vi "Main_Module.vi"(11 "Error_In":errorcluster) -> (15 "Error_Out":errorcluster)   [LabVIEW 2023]
doc: "This is the Main VI that simulates the ADQ system. Captures the data generated in Data acquisition VI and send it to Logger VI to log the Errors."
uses:
  Controls/Current_Limit.ctl
  Controls/Temperature_Limit.ctl
  Controls/DAQ_Data.ctl
  Controls/State_and_Data.ctl
  Controls/Queue_Operation_Select.ctl
  Controls/Notifier_Operation_Select.ctl
panel:
  in  "Logging_Rate":u32=1 caption="Logging Rate"
  in  "Exit":bool
  in  "Acquisition":bool
  in  "Temperature_Limit":T1={"Temperature_High_Limit"=50.0, "Temperature_Low_Limit"=30.0} caption="Temperature Limit" {"Temperature_Low_Limit" min=30.0 max=49.0; "Temperature_High_Limit" min=31.0 max=50.0}
  in  "Current_Limit":T2={"Current_High_Limit"=120.0, "Current_Low_Limit"=100.0} caption="Current Limit" {"Current_High_Limit" min=101.0 max=120.0; "Current_Low_Limit" min=100.0 max=119.0}
  out "Temperature":dbl
  out "Current":dbl
  out "Generated_Data":dbl[][](graph)
  # "DAQ System"
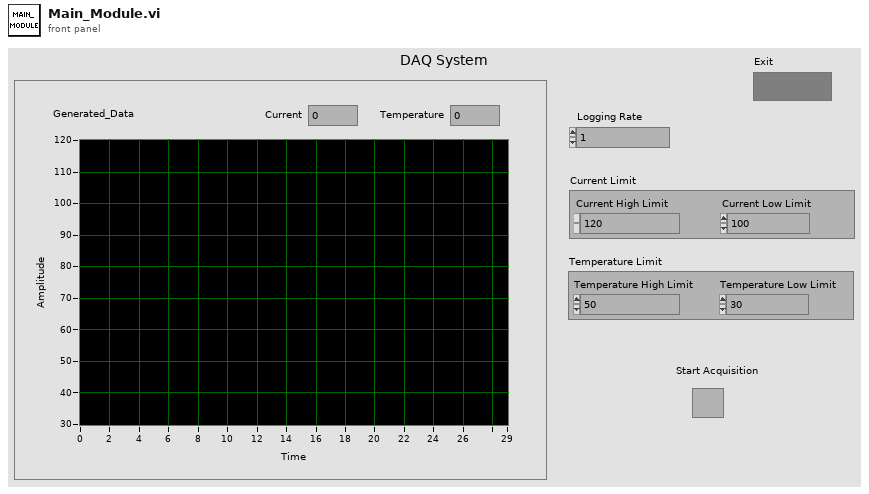
[diagram p1: front panel]
types:
  T1 = typedef "Temperature_Limit.ctl" = cluster{"Temperature_High_Limit":dbl, "Temperature_Low_Limit":dbl}
  T2 = typedef "Current_Limit.ctl" = cluster{"Current_High_Limit":dbl, "Current_Low_Limit":dbl}
  T3 = typedef "Queue_Operation_Select.ctl" = enum16{"Obtain_Queue", "Enqueue", "Enqueue_First", "Enqueue_N", "Lossy_Enqueue", "Preview", "Queue_Status", "Dequeue", "Flush", "Release_Queue"}
  T4 = typedef "Notifier_Operation_Select.ctl" = enum16{"Obtain_Notifier", "Send_Notification", "Get_Notifier_Status", "Release_Notifier"}
  T5 = typedef "State_and_Data.ctl" = cluster{"State":string, "Data":variant}
  T6 = typedef "DAQ_Data.ctl" = cluster{"Wait_Time":dbl, "Start/Stop_Acquisition ":bool, "Generated_Data ":dbl[][], "Current":dbl, "Temperature":dbl, "Disabled":enum8{"Enabled", "Disabled", "Disabled and Grayed Out"}, "Temperature_Limit":T1, "Current_Limit":T2, "State_and_Data_In":T5}
  T7 = enum8{"Enabled", "Disabled", "Disabled and Grayed Out"}
  T8 = typedef "Generated_data.ctl" = cluster{"Current_Data":dbl, "Temp_Data":dbl}
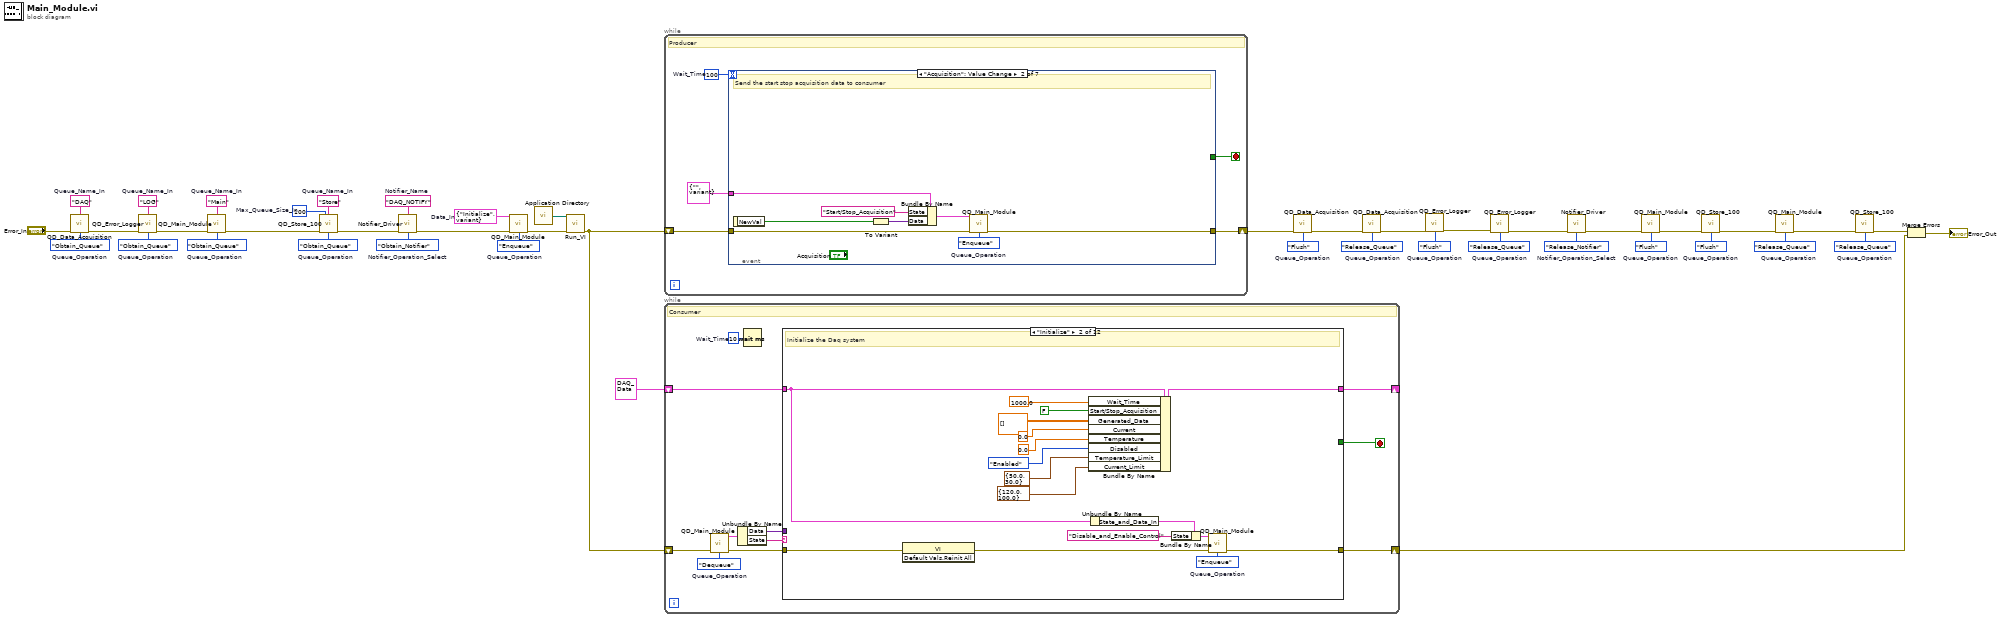
[diagram p0: block diagram]
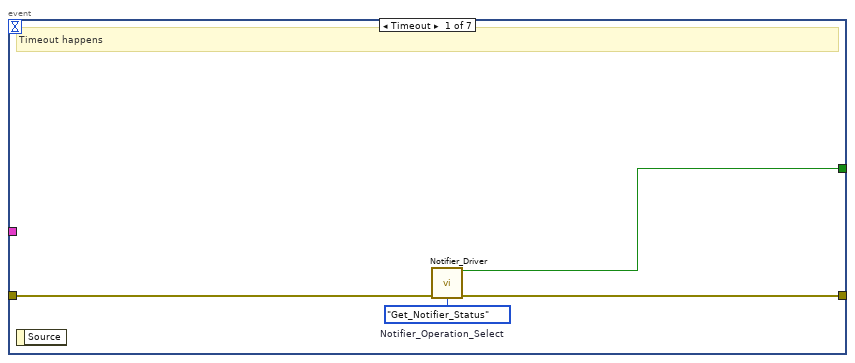
[diagram p2: hidden frame]
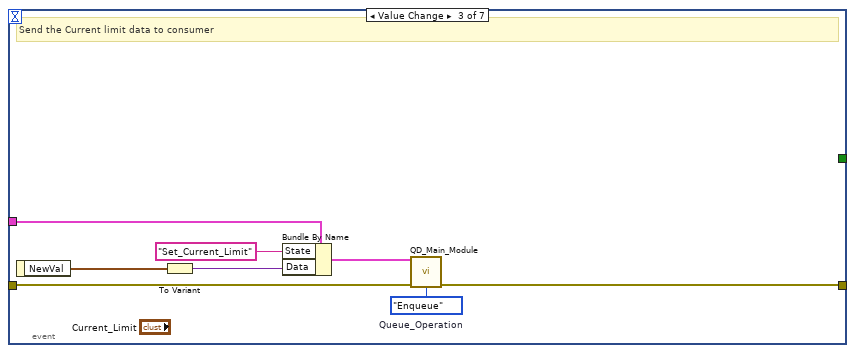
[diagram p3: hidden frame]
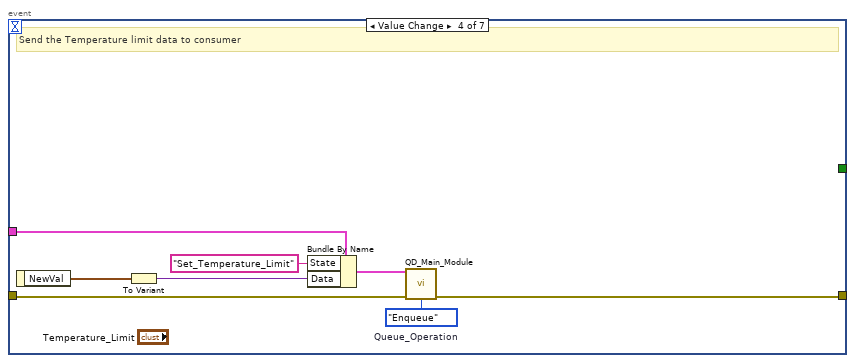
[diagram p4: hidden frame]
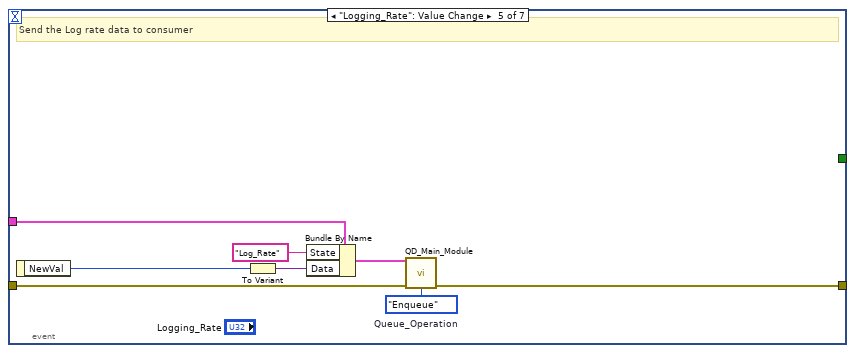
[diagram p5: hidden frame]
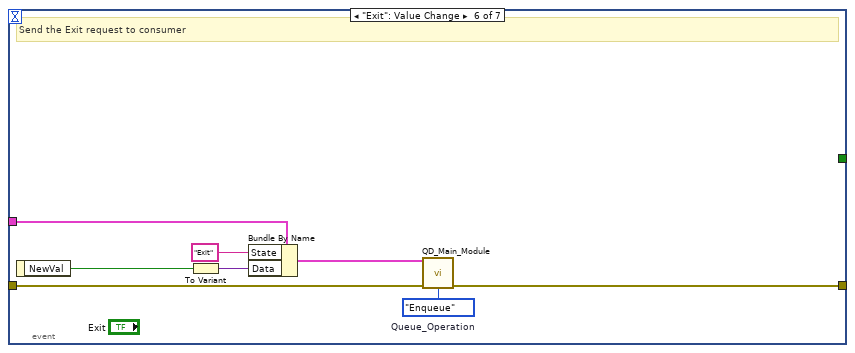
[diagram p6: hidden frame]
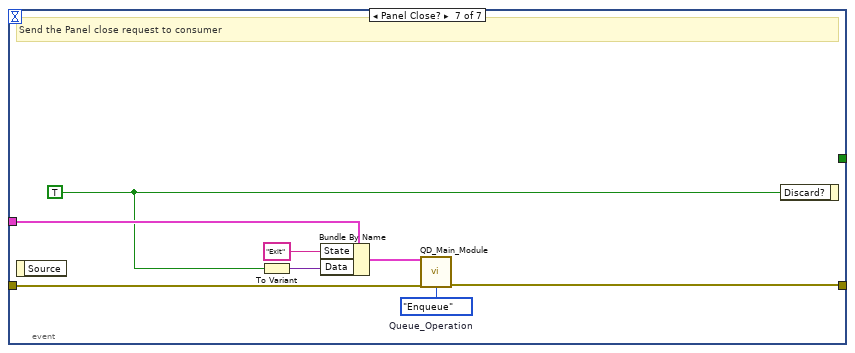
[diagram p7: hidden frame]
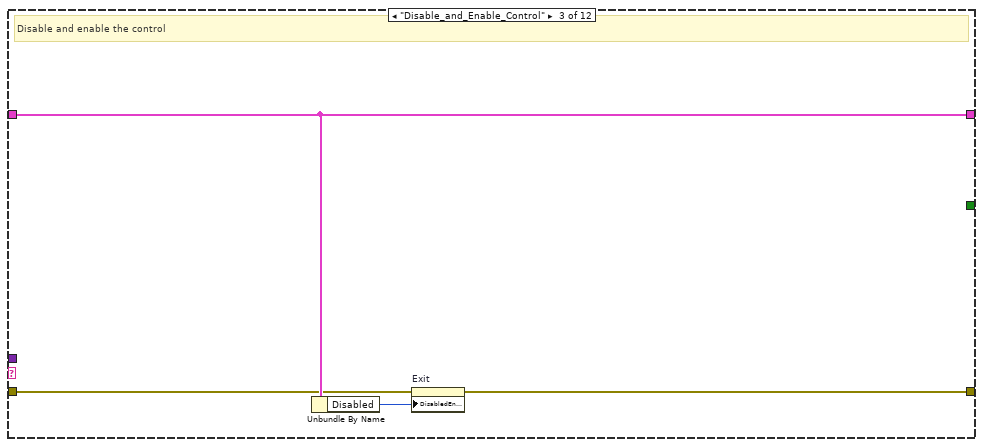
[diagram p9: hidden frame]
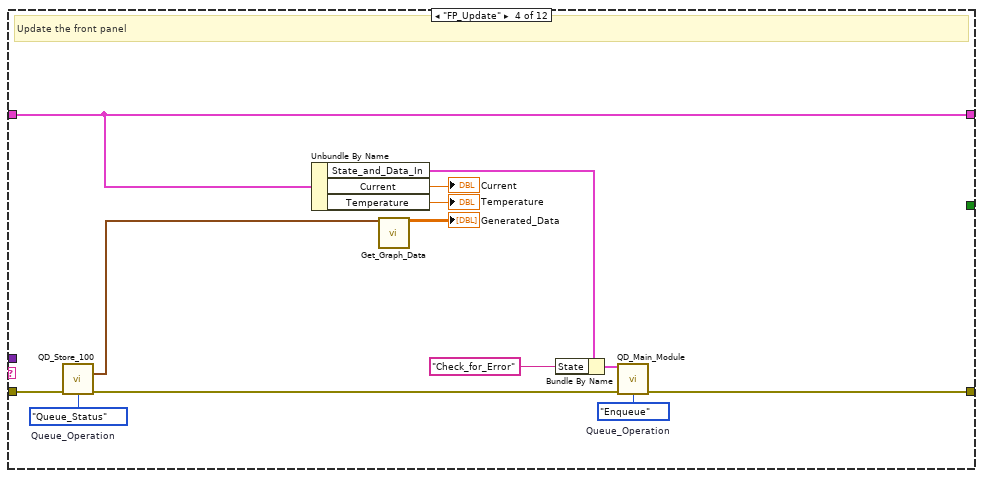
[diagram p10: hidden frame]
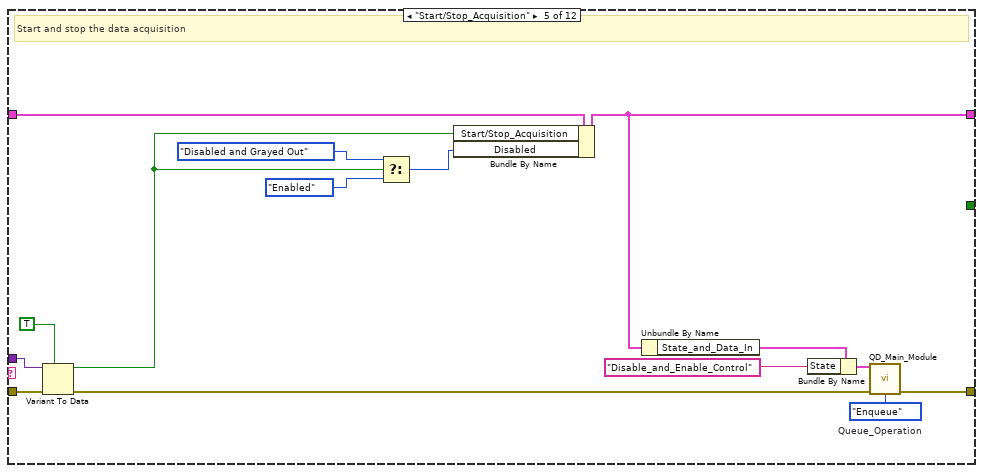
[diagram p11: hidden frame]
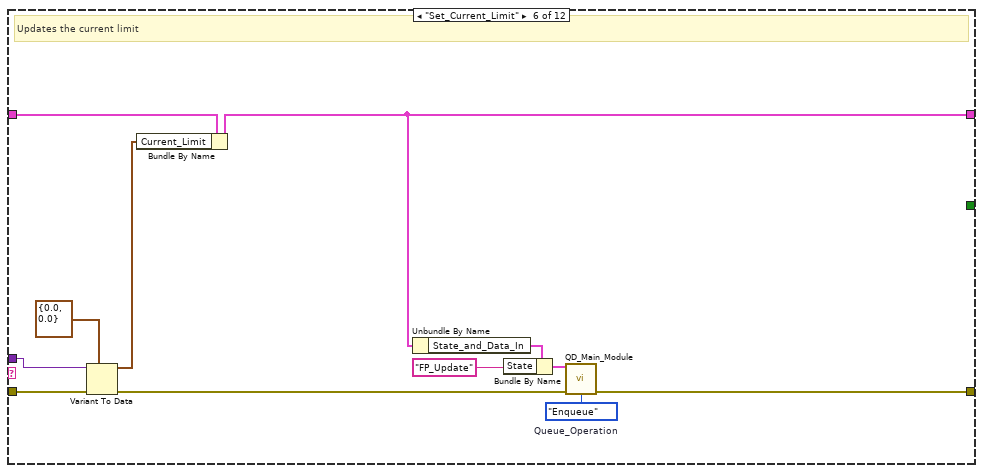
[diagram p12: hidden frame]
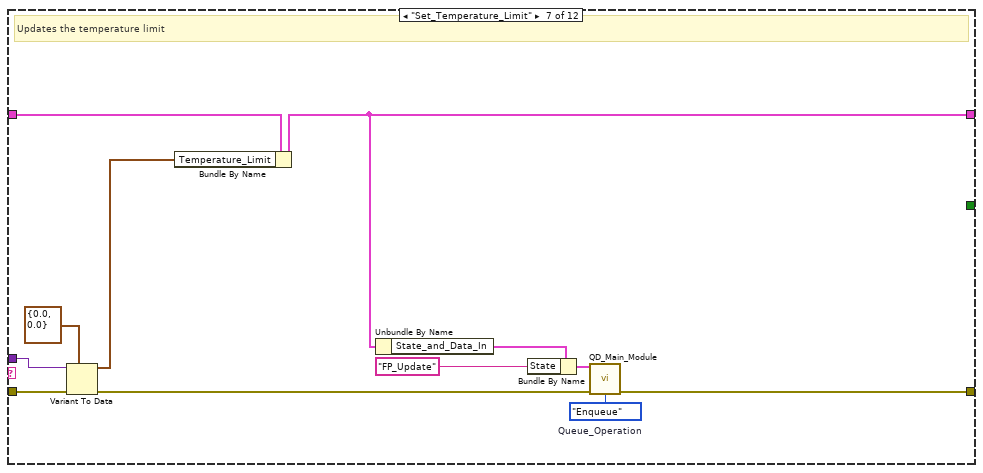
[diagram p13: hidden frame]
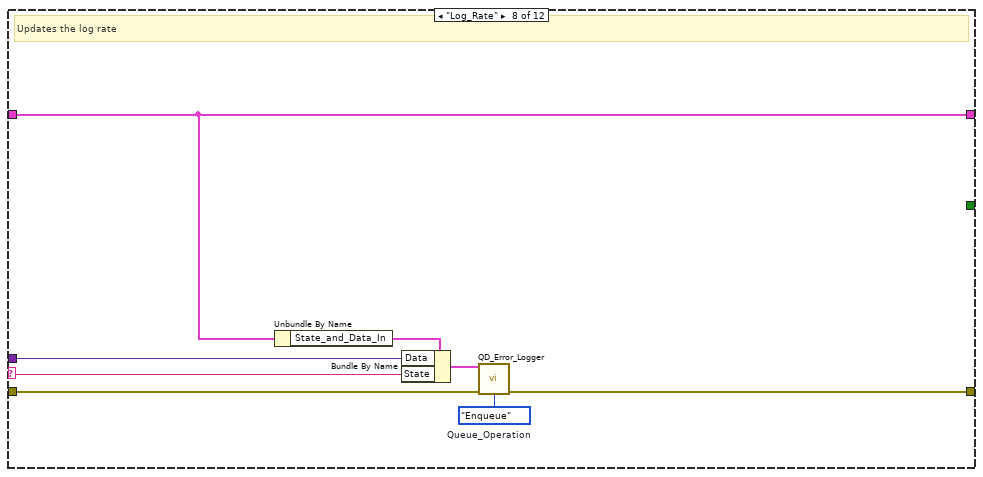
[diagram p14: hidden frame]
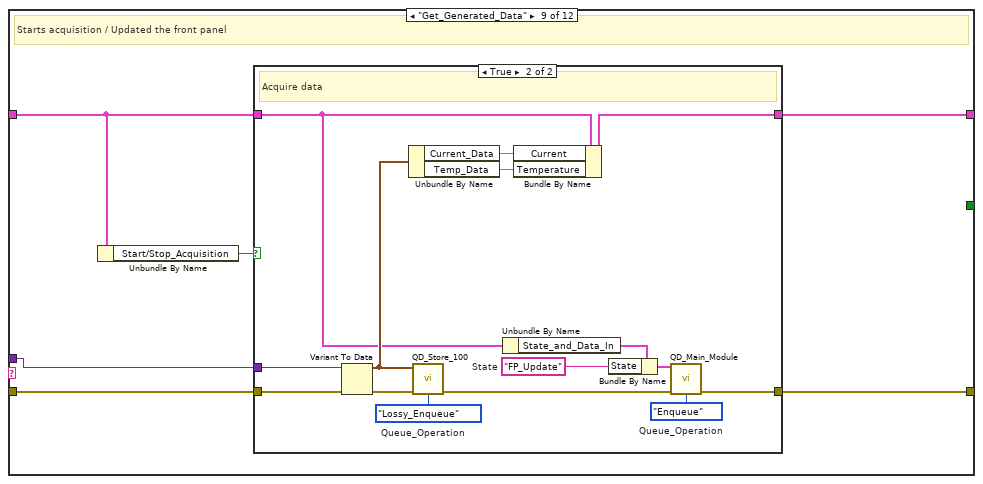
[diagram p15: hidden frame]
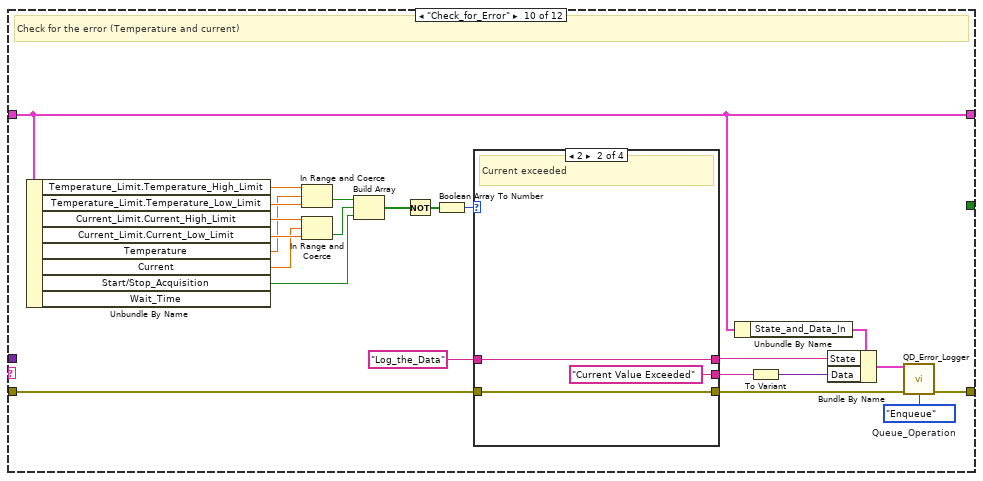
[diagram p17: hidden frame]
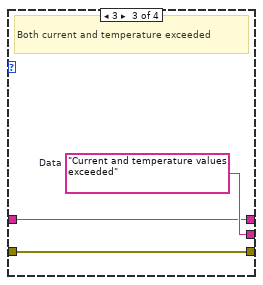
[diagram p19: hidden frame]
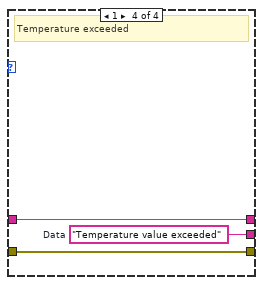
[diagram p20: hidden frame]
diagram:
  w3 = Queue_Operation_Select."Release_Queue"  # Queue_Operation
  w4 = Queue_Operation_Select."Flush"  # Queue_Operation
  w5 = "DAQ_NOTIFY"  # Notifier_Name
  w14 = Notifier_Operation_Select."Release_Notifier"  # Notifier_Operation_Select
  w15 = Queue_Operation_Select."Flush"  # Queue_Operation
  w16 = Queue_Operation_Select."Flush"  # Queue_Operation
  w17 = Queue_Operation_Select."Release_Queue"  # Queue_Operation
  w18 = Queue_Operation_Select."Release_Queue"  # Queue_Operation
  w20 = Queue_Operation_Select."Release_Queue"  # Queue_Operation
  w21 = Queue_Operation_Select."Flush"  # Queue_Operation
  w22 = Notifier_Operation_Select."Obtain_Notifier"  # Notifier_Operation_Select
  w24 = T5 {"State"="Initialize", "Data"=variant}  # Data_In
  w27 = Queue_Operation_Select."Enqueue"  # Queue_Operation
  w29 = "Store"  # Queue_Name_In
  w30 = "Main"  # Queue_Name_In
  w31 = Queue_Operation_Select."Obtain_Queue"  # Queue_Operation
  w33 = "LOG"  # Queue_Name_In
  w34 = "DAQ"  # Queue_Name_In
  w40 = Queue_Operation_Select."Obtain_Queue"  # Queue_Operation
  w41 = Queue_Operation_Select."Obtain_Queue"  # Queue_Operation
  w38 = 100  # Max_Queue_Size_In
  w43 = Queue_Operation_Select."Obtain_Queue"  # Queue_Operation
  n1 = call "QD_Data_Acquisition.vi"("Queue_Name_In"=w34, "Error_In"="Error_In", "Queue_Operation"=w43) -> ("Error_Out"=w44:errorcluster)  [unwired: 10 in, 2 out]
  n2 = call "QD_Error_Logger.vi"("Queue_Name_In"=w33, "Error_In"=w44, "Queue_Operation"=w41) -> ("Error_Out"=w42:errorcluster)  [unwired: 11 in, 1 out]
  n3 = call "QD_Main_Module.vi"("Queue_Name_In"=w30, "Error_In"=w42, "Queue_Operation"=w31) -> ("Error_Out"=w32:errorcluster)  [unwired: 10 in, 2 out]
  n4 = call "QD_Store_100.vi"("Max_Queue_Size_In"=w38, "Queue_Name_In"=w29, "Error_In"=w32, "Queue_Operation"=w40) -> ("Error_Out"=w37:errorcluster)  [unwired: 9 in, 2 out]
  n5 = call "Notifier_Driver.vi"("Notifier_Name"=w5, "Error_In"=w37, "Notifier_Operation_Select"=w22) -> ("Error_Out"=w23:errorcluster)  [unwired: 11 in, 1 out]
  n6 = call "QD_Main_Module.vi"("Data_In"=w24, "Error_In"=w23, "Queue_Operation"=w27) -> ("Error_Out"=w28:errorcluster)  [unwired: 10 in, 2 out]
  n7 = call <vilib>:"Application Directory.vi"() -> ("Application Directory"=w39:path)
  n8 = call "Run_VI.vi"("Application_Directory"=w39, "Error_In"=w28) -> ("Error_Out"=w26:errorcluster)  [unwired: 13 in]
  n9 = while {
    shift-right: [w55] -> _
    shift-left: T6 {"Wait_Time"=1000.0, "Start/Stop_Acquisition "=FALSE, "Generated_Data "=[], "Current"=0.0, "Temperature"=0.0, "Disabled"=enum."Enabled", "Temperature_Limit"={"Temperature_High_Limit"=0.0, "Temperature_Low_Limit"=0.0}, "Current_Limit"={"Current_High_Limit"=101.0, "Current_Low_Limit"=100.0}, "State_and_Data_In"={"State"="", "Data"=variant}} -> [w47]
    shift-right: [w45] -> w25
    shift-left: w26 -> [w54]
    stop <- w48 stop-if-true
    w46 = u32 10  # Wait_Time
    w52 = Queue_Operation_Select."Dequeue"  # Queue_Operation
    # "Consumer"
    n10 = call "QD_Main_Module.vi"("Error_In"=w54, "Queue_Operation"=w52) -> ("Data_Out"=w51:T5, "Error_Out"=w53:errorcluster)  [unwired: 11 in, 1 out]
    n11 = Unbundle By Name(w51) -> ("Data"=w49:variant, "State"=w50:string)
    n12 = Wait (ms)(milliseconds to wait=w46) -> ()  [unwired: 1 out]
    n13 = case shown="\"Initialize\"" w50 {
      selector: w50 -> [_ _ _ _ _ _ _ w135 _ _ _ _]
      tunnel: w53 -> [w56 w74 w77 w85 w106 w118 w130 w138 w144 w171 w204 w224]
      tunnel: w47 -> [w57 w61 w78 w91 w96 w111 w123 w133 w142 w164 w197 w225]
      tunnel: [w57 w73 w78 w91 w92 w110 w121 w133 w140 w164 w197 w225] -> w55
      tunnel: w49 -> [_ _ _ _ w105 w117 w129 w137 w143 _ _ _]
      tunnel: [_ _ _ _ _ _ _ _ _ _ _ w215] -> w48
      tunnel: [w56 w58 w75 w79 w93 w107 w119 w131 w139 w162 w195 w214] -> w45
      frame Default {
        # "Nothing will be done here"
      }
      frame "Initialize" {
        w64 = Queue_Operation_Select."Enqueue"  # Queue_Operation
        # "Initialize the Daq system"
        n14 = invoke class="VI" method="Default Vals.Reinit All"(error in=w74) -> (error out=w62:errorcluster)  [unwired: 2 in, 2 out]
        n15 = Bundle By Name(cluster=w61, "Wait_Time"=1000.0, "Start/Stop_Acquisition"=FALSE, "Generated_Data"=dbl[][] [], "Current"=0.0, "Temperature"=0.0, "Disabled"=T7."Enabled", "Temperature_Limit"=T1 {"Temperature_High_Limit"=50.0, "Temperature_Low_Limit"=30.0}, "Current_Limit"=T2 {"Current_High_Limit"=120.0, "Current_Low_Limit"=100.0}) -> (w73:T6)
        n16 = Unbundle By Name(w61) -> ("State_and_Data_In"=w60:T5)
        n17 = Bundle By Name(cluster=w60, "State"="Disable_and_Enable_Control") -> (w63:T5)
        n18 = call "QD_Main_Module.vi"("Data_In"=w63, "Error_In"=w62, "Queue_Operation"=w64) -> ("Error_Out"=w58:errorcluster)  [unwired: 10 in, 2 out]
      }
      frame "Disable_and_Enable_Control" {
        # "Disable and enable the control"
        n19 = Unbundle By Name(w78) -> ("Disabled"=w76:T7)
        n20 = property on="Exit" class="Bool (strict)"(error in=w77, "DisabledEnum"=w76) -> (error out=w75:errorcluster)  [unwired: 1 in, 1 out]
      }
      frame "FP_Update" {
        w84 = Queue_Operation_Select."Enqueue"  # Queue_Operation
        w88 = Queue_Operation_Select."Queue_Status"  # Queue_Operation
        # "Update the front panel"
        n21 = call "QD_Store_100.vi"("Error_In"=w85, "Queue_Operation"=w88) -> ("Total_Data"=w86:T8[], "Error_Out"=w82:errorcluster)  [unwired: 11 in, 1 out]
        n22 = Unbundle By Name(w91) -> ("State_and_Data_In"=w81:T5, "Current"=→"Current":dbl, "Temperature"=→"Temperature":dbl)
        n23 = call "Get_Graph_Data.vi"("Total_Data"=w86) -> ("Array"=→"Generated_Data":dbl[][])  [unwired: 14 in]
        n24 = Bundle By Name(cluster=w81, "State"="Check_for_Error") -> (w83:T5)
        n25 = call "QD_Main_Module.vi"("Data_In"=w83, "Error_In"=w82, "Queue_Operation"=w84) -> ("Error_Out"=w79:errorcluster)  [unwired: 10 in, 2 out]
      }
      frame "Start/Stop_Acquisition" {
        w99 = Queue_Operation_Select."Enqueue"  # Queue_Operation
        # "Start and stop the data acquisition"
        n26 = Variant To Data(error in=w106, type=TRUE, Variant=w105) -> (data=w101:bool, error out=w97:errorcluster)
        n27 = Select(t=T7."Disabled and Grayed Out", s=w101, f=T7."Enabled" ("Disabled")) -> (s? t:f=w103:T7)
        n28 = Bundle By Name(cluster=w96, "Start/Stop_Acquisition"=w101, "Disabled"=w103) -> (w92:T6)
        n29 = Unbundle By Name(w92) -> ("State_and_Data_In"=w95:T5)
        n30 = Bundle By Name(cluster=w95, "State"="Disable_and_Enable_Control") -> (w98:T5)
        n31 = call "QD_Main_Module.vi"("Data_In"=w98, "Error_In"=w97, "Queue_Operation"=w99) -> ("Error_Out"=w93:errorcluster)  [unwired: 10 in, 2 out]
      }
      frame "Set_Current_Limit" {
        w112 = Queue_Operation_Select."Enqueue"  # Queue_Operation
        # "Updates the current limit"
        n32 = Variant To Data(error in=w118, type=T2 {"Current_High_Limit"=0.0, "Current_Low_Limit"=0.0} ("Current_Limit"), Variant=w117) -> (data=w115:T2, error out=w113:errorcluster)
        n33 = Bundle By Name(cluster=w111, "Current_Limit"=w115) -> (w110:T6)
        n34 = Unbundle By Name(w110) -> ("State_and_Data_In"=w109:T5)
        n35 = Bundle By Name(cluster=w109, "State"="FP_Update") -> (w114:T5)
        n36 = call "QD_Main_Module.vi"("Data_In"=w114, "Error_In"=w113, "Queue_Operation"=w112) -> ("Error_Out"=w107:errorcluster)  [unwired: 10 in, 2 out]
      }
      frame "Set_Temperature_Limit" {
        w120 = Queue_Operation_Select."Enqueue"  # Queue_Operation
        # "Updates the temperature limit"
        n37 = Variant To Data(error in=w130, type=T1 {"Temperature_High_Limit"=0.0, "Temperature_Low_Limit"=0.0} ("Temperature_Limit"), Variant=w129) -> (data=w127:T1, error out=w125:errorcluster)
        n38 = Bundle By Name(cluster=w123, "Temperature_Limit"=w127) -> (w121:T6)
        n39 = Unbundle By Name(w121) -> ("State_and_Data_In"=w122:T5)
        n40 = Bundle By Name(cluster=w122, "State"="FP_Update") -> (w126:T5)
        n41 = call "QD_Main_Module.vi"("Data_In"=w126, "Error_In"=w125, "Queue_Operation"=w120) -> ("Error_Out"=w119:errorcluster)  [unwired: 10 in, 2 out]
      }
      frame "Log_Rate" {
        w134 = Queue_Operation_Select."Enqueue"  # Queue_Operation
        # "Updates the log rate"
        n42 = Unbundle By Name(w133) -> ("State_and_Data_In"=w132:T5)
        n43 = Bundle By Name(cluster=w132, "Data"=w137, "State"=w135) -> (w136:T5)
        n44 = call "QD_Error_Logger.vi"("State_and_Data_In"=w136, "Error_In"=w138, "Queue_Operation"=w134) -> ("Error_Out"=w131:errorcluster)  [unwired: 11 in, 1 out]
      }
      frame "Get_Generated_Data" {
        # "Starts acquisition / Updated the front panel"
        n45 = Unbundle By Name(w142) -> ("Start/Stop_Acquisition"=w141:bool)
        n46 = case shown="True" w141 {
          tunnel: w144 -> [w145 w160]
          tunnel: w142 -> [w146 w147]
          tunnel: w143 -> [_ w158]
          tunnel: [w146 w156] -> w140
          tunnel: [w145 w148] -> w139
          frame False {
          }
          frame True {
            w152 = Queue_Operation_Select."Enqueue"  # Queue_Operation
            w151 = "FP_Update"  # State
            w161 = Queue_Operation_Select."Lossy_Enqueue"  # Queue_Operation
            # "Acquire data"
            n47 = Variant To Data(error in=w160, Variant=w158) -> (data=w157:T8, error out=w159:errorcluster)  [unwired: 1 in]
            n48 = Unbundle By Name(w157) -> ("Current_Data"=w154:dbl, "Temp_Data"=w155:dbl)
            n49 = call "QD_Store_100.vi"("Generated_Data_In"=w157, "Error_In"=w159, "Queue_Operation"=w161) -> ("Error_Out"=w149:errorcluster)  [unwired: 10 in, 2 out]
            n50 = Unbundle By Name(w147) -> ("State_and_Data_In"=w150:T5)
            n51 = Bundle By Name(cluster=w147, "Current"=w154, "Temperature"=w155) -> (w156:T6)
            n52 = Bundle By Name(cluster=w150, "State"=w151) -> (w153:T5)
            n53 = call "QD_Main_Module.vi"("Data_In"=w153, "Error_In"=w149, "Queue_Operation"=w152) -> ("Error_Out"=w148:errorcluster)  [unwired: 10 in, 2 out]
          }
        }
      }
      frame "Check_for_Error" {
        w172 = Queue_Operation_Select."Enqueue"  # Queue_Operation
        # "Check for the error (Temperature and current)"
        n54 = Unbundle By Name(w164) -> ("Temperature_Limit.Temperature_High_Limit"=w184:dbl, "Temperature_Limit.Temperature_Low_Limit"=w183:dbl, "Current_Limit.Current_High_Limit"=w182:dbl, "Current_Limit.Current_Low_Limit"=w181:dbl, "Temperature"=w170:dbl, "Current"=w169:dbl, "Start/Stop_Acquisition"=w168:bool)  [unwired: 1 out]
        n55 = In Range and Coerce(upper limit=w184, x=w170, lower limit=w183) -> (In Range?=w166:bool)  [unwired: 1 out]
        n56 = In Range and Coerce(upper limit=w182, x=w169, lower limit=w181) -> (In Range?=w167:bool)  [unwired: 1 out]
        n57 = Build Array(w166, w167, w168) -> (w179:bool[])
        n58 = Not(x=w179) -> (.not. x?=w165:bool[])
        n59 = Boolean Array To Number(Boolean array=w165) -> (number=w178:u32)
        n60 = case shown="2" w178 {
          tunnel: [w185 w188 w191 w194] -> w180
          tunnel: w171 -> [w185 w188 w191 w194]
          tunnel: [_ "Current Value Exceeded" ("Data") w190 w193] -> w177
          tunnel: [_ w186 w189 w192] -> w174
          tunnel: "Log_the_Data" ("State") -> [_ w186 w189 w192]
          frame 0, Default {
          }
          frame 2 {
            # "Current exceeded"
          }
          frame 3 {
            w190 = "Current and temperature values exceeded"  # Data
            # "Both current and temperature exceeded"
          }
          frame 1 {
            w193 = "Temperature value exceeded"  # Data
            # "Temperature exceeded"
          }
        }
        n61 = Unbundle By Name(w164) -> ("State_and_Data_In"=w163:T5)
        n62 = To Variant(anything=w177) -> (Variant=w173:variant)
        n63 = Bundle By Name(cluster=w163, "State"=w174, "Data"=w173) -> (w175:T5)
        n64 = call "QD_Error_Logger.vi"("State_and_Data_In"=w175, "Error_In"=w180, "Queue_Operation"=w172) -> ("Error_Out"=w162:errorcluster)  [unwired: 11 in, 1 out]
      }
      frame "Error" {
        w209 = "%d%s%s"  # Format_String
        w210 = "Application Error"  # Initial_String
        w211 = "Stop"  # T_Button
        w212 = "Continue"  # F_Button
        # "Handles the appplication error"
        n65 = Unbundle By Name(w204) -> ("code"=w206:i32, "source"=w205:string)
        n66 = call <vilib>:"Clear Errors.vi"("error in (no error)"=w204) -> ("error out"=w207:errorcluster)  [unwired: 5 in, 1 out]
        n67 = Format Into String(format string=w209, initial string=w210, error in=w207, w206, "\n", w205) -> (resulting string=w213:string, error out=w199:errorcluster)
        n68 = Unbundle By Name(w197) -> ("State_and_Data_In"=w196:T5)
        n69 = Two Button Dialog(message=w213, 1:w212, 2:w211) -> (T button?=w202:bool)
        n70 = Select(t="Exit" ("State"), s=w202, f="") -> (s? t:f=w198:string)
        n71 = Bundle By Name(cluster=w196, "State"=w198) -> (w200:T5)
        n72 = call "QD_Main_Module.vi"("Data_In"=w200, "Error_In"=w199) -> ("Error_Out"=w195:errorcluster)  [unwired: 11 in, 2 out]
      }
      frame "Exit" {
        w218 = Notifier_Operation_Select."Send_Notification"  # Notifier_Operation_Select
        w219 = T5 {"State"="Exit", "Data"=variant}  # State_and_Data_In
        w220 = Queue_Operation_Select."Enqueue_First"  # Queue_Operation
        w221 = Queue_Operation_Select."Enqueue_First"  # Queue_Operation
        # "Exit the Application if the user wants to exit"
        n73 = disable-structure shown="Default" {
          disable-tunnel: [w226 w230] -> w215
          frame condition #0 (active) {
            w227 = "No"  # Back
            w228 = "Yes"  # Stop_Execution
            w229 = "Do you want to Stop the execution"  # Message
            # "Developer_Mode"
            n74 = Two Button Dialog(message=w229, 1:w227, 2:w228) -> (T button?=w226:bool)
          }
          frame condition #1 {
            w230 = TRUE  # Stop?
            # "Run_Time_Mode"
          }
        }
        n75 = Select(t=w219, s=w215, f=T5 {"State"="", "Data"=variant}) -> (s? t:f=w217:T5)
        n76 = call "QD_Error_Logger.vi"("State_and_Data_In"=w217, "Error_In"=w224, "Queue_Operation"=w221) -> ("Error_Out"=w223:errorcluster)  [unwired: 11 in, 1 out]
        n77 = call "QD_Data_Acquisition.vi"("State_and_Data_In"=w217, "Error_In"=w223, "Queue_Operation"=w220) -> ("Error_Out"=w222:errorcluster)  [unwired: 10 in, 2 out]
        n78 = call "Notifier_Driver.vi"("Notification"=w215, "Error_In"=w222, "Notifier_Operation_Select"=w218) -> ("Error_Out"=w214:errorcluster)  [unwired: 11 in, 1 out]
      }
    }
  }
  n79 = while {
    shift-right: [w231] -> w8
    shift-left: w26 -> [w235]
    stop <- w233 stop-if-true
    w234 = 100  # Wait_Time
    # "Producer"
    n80 = event shown="[1] \"Acquisition\": Value Change" {
      selector: _ -> [_ _ _ _ _ _ _]
      dyn-events: _ -> [_ _ _ _ _ _ _]
      timeout: w234 -> [_ _ _ _ _ _ _]
      tunnel: w235 -> [w236 w245 w253 w260 w271 w277 w283]
      tunnel: [w239 w244 w252 w259 w265 w276 w285] -> w231
      tunnel: [w237 _ _ _ _ _ _] -> w233
      tunnel: T5 {"State"="", "Data"=variant} ("Data_In") -> [_ w240 w249 w258 w266 w275 w284]
      event Timeout {
        w238 = Notifier_Operation_Select."Get_Notifier_Status"  # Notifier_Operation_Select
        # "Timeout happens"
        n81 = event-data() -> ()  [unwired: 1 in, 1 out]
        n82 = call "Notifier_Driver.vi"("Error_In"=w236, "Notifier_Operation_Select"=w238) -> ("Latest_Notification"=w237:bool, "Error_Out"=w239:errorcluster)  [unwired: 12 in]
      }
      event "Acquisition": Value Change {
        w243 = Queue_Operation_Select."Enqueue"  # Queue_Operation
        # "Send the start stop acquisition data to consumer"
        n83 = event-data() -> ("NewVal"=w247:bool)  [unwired: 1 in]
        n84 = To Variant(anything=w247) -> (Variant=w241:variant)
        n85 = Bundle By Name(cluster=w240, "State"="Start/Stop_Acquisition", "Data"=w241) -> (w246:T5)
        n86 = call "QD_Main_Module.vi"("Data_In"=w246, "Error_In"=w245, "Queue_Operation"=w243) -> ("Error_Out"=w244:errorcluster)  [unwired: 10 in, 2 out]
      }
      event Value Change {
        w254 = Queue_Operation_Select."Enqueue"  # Queue_Operation
        # "Send the Current limit data to consumer"
        n87 = event-data() -> ("NewVal"=w255:T2)  [unwired: 1 in]
        n88 = To Variant(anything=w255) -> (Variant=w248:variant)
        n89 = Bundle By Name(cluster=w249, "State"="Set_Current_Limit", "Data"=w248) -> (w251:T5)
        n90 = call "QD_Main_Module.vi"("Data_In"=w251, "Error_In"=w253, "Queue_Operation"=w254) -> ("Error_Out"=w252:errorcluster)  [unwired: 10 in, 2 out]
      }
      event Value Change {
        w261 = Queue_Operation_Select."Enqueue"  # Queue_Operation
        # "Send the Temperature limit data to consumer"
        n91 = event-data() -> ("NewVal"=w263:T1)  [unwired: 1 in]
        n92 = To Variant(anything=w263) -> (Variant=w257:variant)
        n93 = Bundle By Name(cluster=w258, "State"="Set_Temperature_Limit", "Data"=w257) -> (w262:T5)
        n94 = call "QD_Main_Module.vi"("Data_In"=w262, "Error_In"=w260, "Queue_Operation"=w261) -> ("Error_Out"=w259:errorcluster)  [unwired: 10 in, 2 out]
      }
      event "Logging_Rate": Value Change {
        w268 = Queue_Operation_Select."Enqueue"  # Queue_Operation
        # "Send the Log rate data to consumer"
        n95 = event-data() -> ("NewVal"=w264:u32)  [unwired: 1 in]
        n96 = To Variant(anything=w264) -> (Variant=w269:variant)
        n97 = Bundle By Name(cluster=w266, "State"="Log_Rate", "Data"=w269) -> (w270:T5)
        n98 = call "QD_Main_Module.vi"("Data_In"=w270, "Error_In"=w271, "Queue_Operation"=w268) -> ("Error_Out"=w265:errorcluster)  [unwired: 10 in, 2 out]
      }
      event "Exit": Value Change {
        w272 = Queue_Operation_Select."Enqueue"  # Queue_Operation
        # "Send the Exit request to consumer"
        n99 = event-data() -> ("NewVal"=w279:bool)  [unwired: 1 in]
        n100 = To Variant(anything=w279) -> (Variant=w273:variant)
        n101 = Bundle By Name(cluster=w275, "State"="Exit", "Data"=w273) -> (w278:T5)
        n102 = call "QD_Main_Module.vi"("Data_In"=w278, "Error_In"=w277, "Queue_Operation"=w272) -> ("Error_Out"=w276:errorcluster)  [unwired: 10 in, 2 out]
      }
      event Panel Close? {
        w287 = Queue_Operation_Select."Enqueue"  # Queue_Operation
        w280 = TRUE ("Discard?")
        # "Send the Panel close request to consumer"
        n103 = event-data() -> ()  [unwired: 1 in, 1 out]
        n104 = To Variant(anything=w280) -> (Variant=w281:variant)
        n105 = Bundle By Name(cluster=w284, "State"="Exit", "Data"=w281) -> (w286:T5)
        n106 = call "QD_Main_Module.vi"("Data_In"=w286, "Error_In"=w283, "Queue_Operation"=w287) -> ("Error_Out"=w285:errorcluster)  [unwired: 10 in, 2 out]
        n107 = event-data("Discard?"=w280) -> ()  [unwired: 1 in, 1 out]
      }
    }
  }
  n108 = call "QD_Data_Acquisition.vi"("Error_In"=w8, "Queue_Operation"=w21) -> ("Error_Out"=w19:errorcluster)  [unwired: 11 in, 2 out]
  n109 = call "QD_Data_Acquisition.vi"("Error_In"=w19, "Queue_Operation"=w3) -> ("Error_Out"=w2:errorcluster)  [unwired: 11 in, 2 out]
  n110 = call "QD_Error_Logger.vi"("Error_In"=w2, "Queue_Operation"=w4) -> ("Error_Out"=w1:errorcluster)  [unwired: 12 in, 1 out]
  n111 = call "QD_Error_Logger.vi"("Error_In"=w1, "Queue_Operation"=w20) -> ("Error_Out"=w9:errorcluster)  [unwired: 12 in, 1 out]
  n112 = call "Notifier_Driver.vi"("Error_In"=w9, "Notifier_Operation_Select"=w14) -> ("Error_Out"=w13:errorcluster)  [unwired: 12 in, 1 out]
  n113 = call "QD_Main_Module.vi"("Error_In"=w13, "Queue_Operation"=w16) -> ("Error_Out"=w12:errorcluster)  [unwired: 11 in, 2 out]
  n114 = call "QD_Store_100.vi"("Error_In"=w12, "Queue_Operation"=w15) -> ("Error_Out"=w11:errorcluster)  [unwired: 11 in, 2 out]
  n115 = call "QD_Main_Module.vi"("Error_In"=w11, "Queue_Operation"=w18) -> ("Error_Out"=w10:errorcluster)  [unwired: 11 in, 2 out]
  n116 = call "QD_Store_100.vi"("Error_In"=w10, "Queue_Operation"=w17) -> ("Error_Out"=w7:errorcluster)  [unwired: 11 in, 2 out]
  n117 = Merge Errors(w7, w25) -> (→"Error_Out":errorcluster)
